vi "Set Log Thresholds.vi"(8 "error in":errorcluster, 10 "log thresholds":T1 {"Segment Files By" items=["Time", "Size"]}, 11 "logging ref":T2=18446744073709551615 format="%.0x") -> (0 "error out":errorcluster, 3 "logging ref out":T2 format="%.0x")   [LabVIEW 2020, in "AIM ARINC 664 Scripting.lvlib"]
uses:
  AIM ARINC 664 Scripting.lvlib
  <vilib>/NI VeriStand/Custom Device API/Custom Device Item Ref.ctl
  Shared/loggingThreshold_types.ctl
  <vilib>/NI VeriStand/Custom Device API/Custom Device API.lvlib
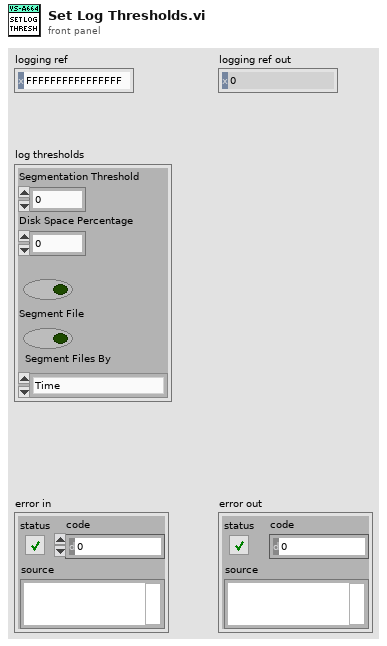
[diagram p1: front panel]
types:
  T1 = typedef "loggingThreshold_types.ctl" = cluster{"Segmentation Threshold":dbl, "Disk Space Percentage":dbl, "Check Disk Space":bool, "Segment File":bool, "Segment Files By":u16}
  T2 = typedef "Custom Device API.lvlib/Custom Device Item Ref.ctl" = u64
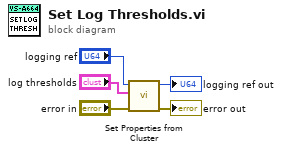
[diagram p0: block diagram]
diagram:
  n1 = call "Set Properties from Cluster.vi"("error in"="error in", "Variant Cluster"="log thresholds", "item ref in"="logging ref") -> ("error out"=→"error out":errorcluster, "item ref out"=→"logging ref out":T2)  [unwired: 7 in]
